vi "JSON to SHW file.vi"(8 "error in (no error)":errorcluster, 10 "Capabilities JSON In":string, 11 "device":string) -> (0 "error out":errorcluster, 2 "SLSC Switch Info":refnum<class "Relay.lvclass">[](array[class]), 3 "SHW Path Out":path)   [LabVIEW 2015, in "SLSC Switch.lvlib" / "SLSC Switch.lvclass"]
uses:
  SLSC Switch.lvclass
  Relay/Relay.lvclass
  Controls/JSON.Relay.ctl
  Controls/JSON.RelaySLSCAction.ctl
  Relay/Property.ctl
  Relay/Command.ctl
  <vilib>/Utility/config.llb/Write Key (I32).vi
  <vilib>/Utility/config.llb/NI_LVConfig.lvlib
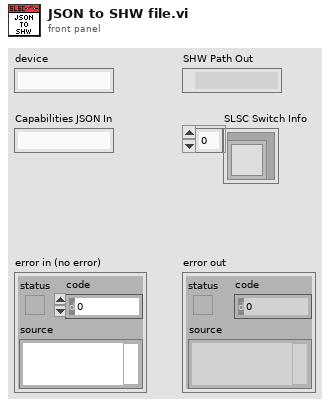
[diagram p1: front panel]
types:
  T1 = typedef "JSON.Relay.ctl" = cluster{"name":string, "actions":T2[]}
  T2 = typedef "JSON.RelaySLSCAction.ctl" = cluster{"type":string, "resource":string, "value":string}
  T3 = typedef "SLSC Switch.lvlib/Relay.lvclass/Property.ctl" = cluster{"resource name":string, "property":refnum<k21>}
  T4 = typedef "SLSC Switch.lvlib/Relay.lvclass/Command.ctl" = cluster{"resource name":string, "command":refnum<k21>}
  T5 = typedef "NI_LVConfig.lvlib/Config Data RefNum.ctl" = refnum<k1>
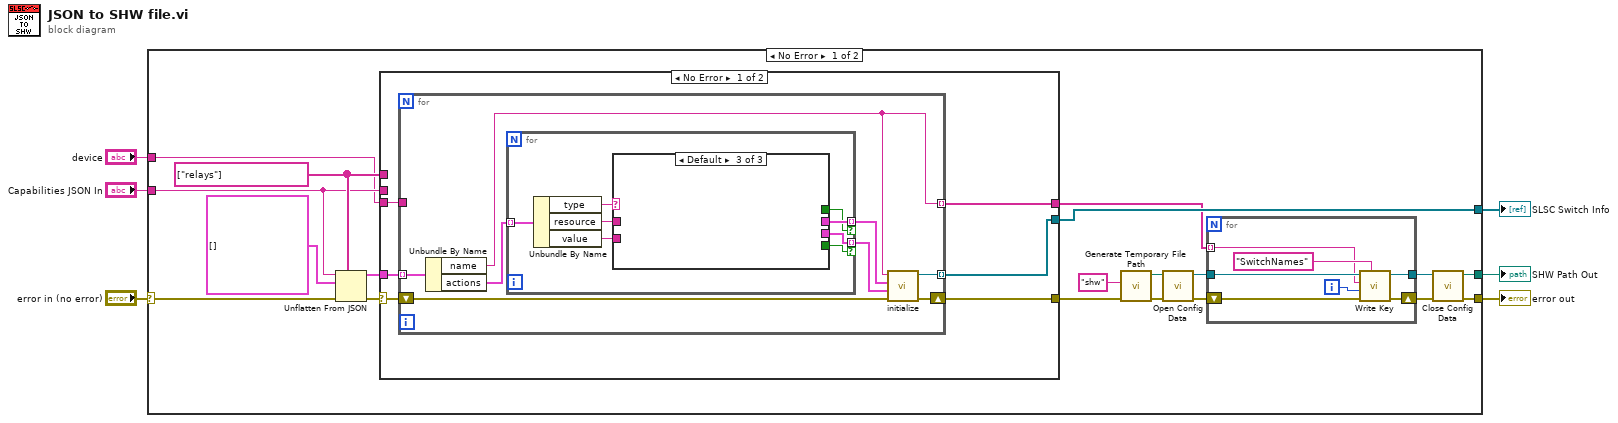
[diagram p0: block diagram]
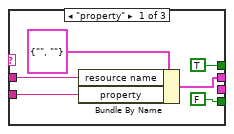
[diagram p2: hidden frame]
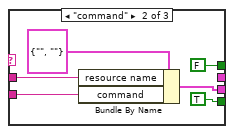
[diagram p3: hidden frame]
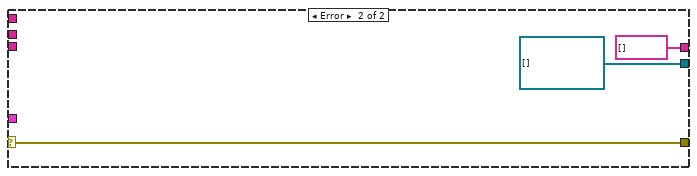
[diagram p4: hidden frame]
diagram:
  n1 = case shown="No Error" "error in (no error)" {
    selector: "error in (no error)" -> [w25 w70]
    tunnel: [w18 w70] -> w5
    tunnel: "Capabilities JSON In" -> [w10 _]
    tunnel: [w16 _] -> w3
    tunnel: "device" -> [w8 _]
    tunnel: [w13 _] -> w1
    frame No Error {
      w11 = string[] ["relays"] ("path")
      n2 = Unflatten From JSON(path=w11, JSON string=w10, type and defaults=T1[] [] ("Array"), error in (no error)=w25) -> (value=w14:T1[], error out=w15:errorcluster)  [unwired: 3 in]
      n3 = case shown="No Error" w15 {
        selector: w15 -> [w28 w62]
        tunnel: w14 -> [w31 _]
        tunnel: [w30 string[] []] -> w9
        tunnel: [w29 refnum<class "Relay.lvclass">[] []] -> w13
        tunnel: [w27 w62] -> w12
        tunnel: w11 -> [_ _]
        tunnel: w10 -> [_ _]
        tunnel: w8 -> [w26 _]
        frame No Error {
          n4 = for {
            tunnel: w31 -> [w36] mode=indexing
            tunnel: [w34] -> w30 mode=indexing
            tunnel: [w39] -> w29 mode=indexing
            shift-right: [w37] -> w27
            shift-left: w28 -> [w38]
            tunnel: w26 -> [_]
            n5 = Unbundle By Name(w36) -> ("name"=w34:string, "actions"=w35:T2[])
            n6 = for {
              tunnel: w35 -> [w47] mode=indexing
              tunnel: [w43] -> w33 mode=indexing if=w41
              tunnel: [w42] -> w32 mode=indexing if=w40
              n7 = Unbundle By Name(w47) -> ("type"=w46:string, "resource"=w45:string, "value"=w44:string)
              n8 = case shown="Default" w46 {
                tunnel: w45 -> [w52 w59 _]
                tunnel: w44 -> [w51 w58 _]
                tunnel: [w50 _ _] -> w43
                tunnel: [TRUE FALSE _] -> w41
                tunnel: [_ w55 _] -> w42
                tunnel: [FALSE TRUE _] -> w40
                frame "property" {
                  n9 = Bundle By Name(cluster=T3 {"resource name"="", "property"=""} ("Property"), "resource name"=w52, "property"=w51) -> (w50:T3)
                }
                frame "command" {
                  n10 = Bundle By Name(cluster=T4 {"resource name"="", "command"=""} ("Command"), "resource name"=w59, "command"=w58) -> (w55:T4)
                }
                frame Default {
                }
              }
            }
            n11 = call "initialize.vi"("error in (no error)"=w38, "Commands"=w32, "Properties"=w33, "name"=w34) -> ("error out"=w37:errorcluster, "Relay out"=w39:refnum<class "Relay.lvclass">)  [unwired: 6 in]
          }
        }
        frame Error {
        }
      }
      n12 = call <vilib>:"Generate Temporary File Path.vi"("error in (no error)"=w12, "Temporary File Extension (tmp)"="shw") -> ("error out"=w23:errorcluster, "Unique Temporary File Path"=w17:path)  [unwired: 8 in]
      n13 = call <vilib>:"Open Config Data.vi"("error in (no error)"=w23, "configuration file path"=w17) -> ("error out"=w21:errorcluster, "refnum"=w22:T5)  [unwired: 7 in, 1 out]
      n14 = for {
        tunnel: w22 -> [w69]
        tunnel: [w68] -> w19
        shift-right: [w66] -> w20
        shift-left: w21 -> [w67]
        tunnel: w9 -> [w63] mode=indexing
        i -> [w64]
        n15 = call-poly <vilib>:"Write Key.vi"("section"="SwitchNames", "error in (no error)"=w67, "value"=w64, "key"=w63, "refnum"=w69) -> ("error out"=w66:errorcluster, "refnum out"=w68:T5)  [unwired: 4 in, 1 out]
      }
      n16 = call <vilib>:"Close Config Data.vi"("error in (no error)"=w20, "refnum"=w19) -> ("error out"=w18:errorcluster, "file path"=w16:path)  [unwired: 8 in]
    }
    frame Error {
    }
  }
  "error out" <- w5
  "SHW Path Out" <- w3
  "SLSC Switch Info" <- w1
